vi "read config.vi"(8 "error in (no error)":errorcluster, 10 "config file path":path, 11 "USB DAQ in":refnum<class "USB DAQ.lvclass">) -> (0 "error out":errorcluster, 3 "USB DAQ out":refnum<class "USB DAQ.lvclass">)   [LabVIEW 2025, in "USB DAQ.lvclass"]
uses:
  USB DAQ.lvclass
  USB DAQ.lvclass/USB DAQ.ctl
  cd2e1b48-1307-4e7b-810b-a5777d732a1e.vi
  <vilib>/JDP Science/JSONtext/JSON text to Variant.vi
  <vilib>/JDP Science/JSONtext/LVClass Serializer/JSONtext LVClass Serializer.lvclass
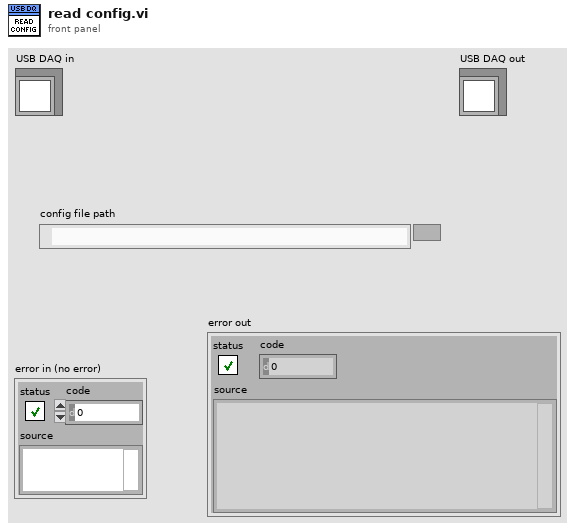
[diagram p1: front panel]
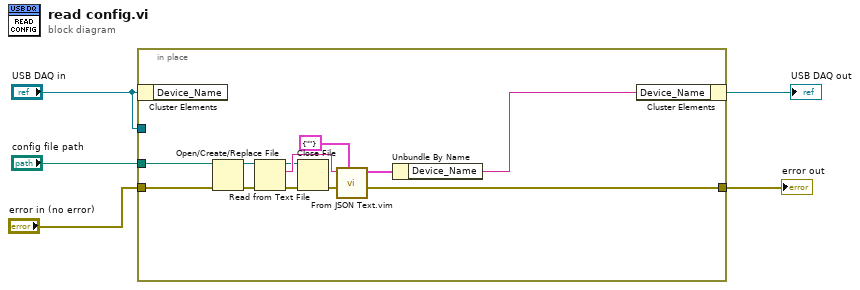
[diagram p0: block diagram]
diagram:
  n1 = in-place {
    in-place-border: "config file path" -> [w11]
    in-place-border: "error in (no error)" -> [w10]
    in-place-border: [w9] -> w3
    in-place-border: "USB DAQ in" -> [_]
    n2 = in-place-cluster #1("USB DAQ in") -> ()  [unwired: 1 out]
    n3 = Open/Create/Replace File(file path (use dialog)=w11, error in=w10) -> (refnum out=w15:refnum<file>, error out=w12:errorcluster)  [unwired: 4 in, 1 out]
    n4 = Read from Text File(file (use dialog)=w15, error in=w12) -> (refnum out=w14:refnum<file>, text=w16:string, error out=w13:errorcluster)  [unwired: 2 in, 1 out]
    n5 = Close File(refnum=w14, error in=w13) -> (error out=w17:errorcluster)  [unwired: 1 out]
    n6 = call "From JSON Text.vim"("Data Type and Default Value"=cluster{"Device_Name":string} {"Device_Name"=""}, "error in (no error)"=w17, "JSON"=w16) -> ("error out"=w9:errorcluster, "Data out"=w7:cluster{"Device_Name":string})  [unwired: 7 in]
    n7 = Unbundle By Name(w7) -> ("Device_Name"=w6:string)
    n8 = in-place-cluster #1("Device_Name"=w6) -> (→"USB DAQ out":refnum<class "USB DAQ.lvclass">)
  }
  "error out" <- w3
